vi "IO配置检测.vi"(7 "错误输入（无错误）":errorcluster, 8 "配置检索操作":T11, 9 "点动轴选择":T10=enum."出料轴", 10 "输出控制":T6, 11 "输入读取":T1) -> (0 "输出配置提取集合":T12, 1 "输入配置提取集合":T12, 3 "轴名称数组":string[](array[string]), 5 "error out":errorcluster)   [LabVIEW 2017]
panel:
  in  "选项卡控件":enum32{"选项卡 1", "选项卡 2", "选项卡 3"}(tab)
  out "轴信息检索list":string[](array[string])
  out "Input检索list":string[](array[string])
  out "Output检索list":string[](array[string])
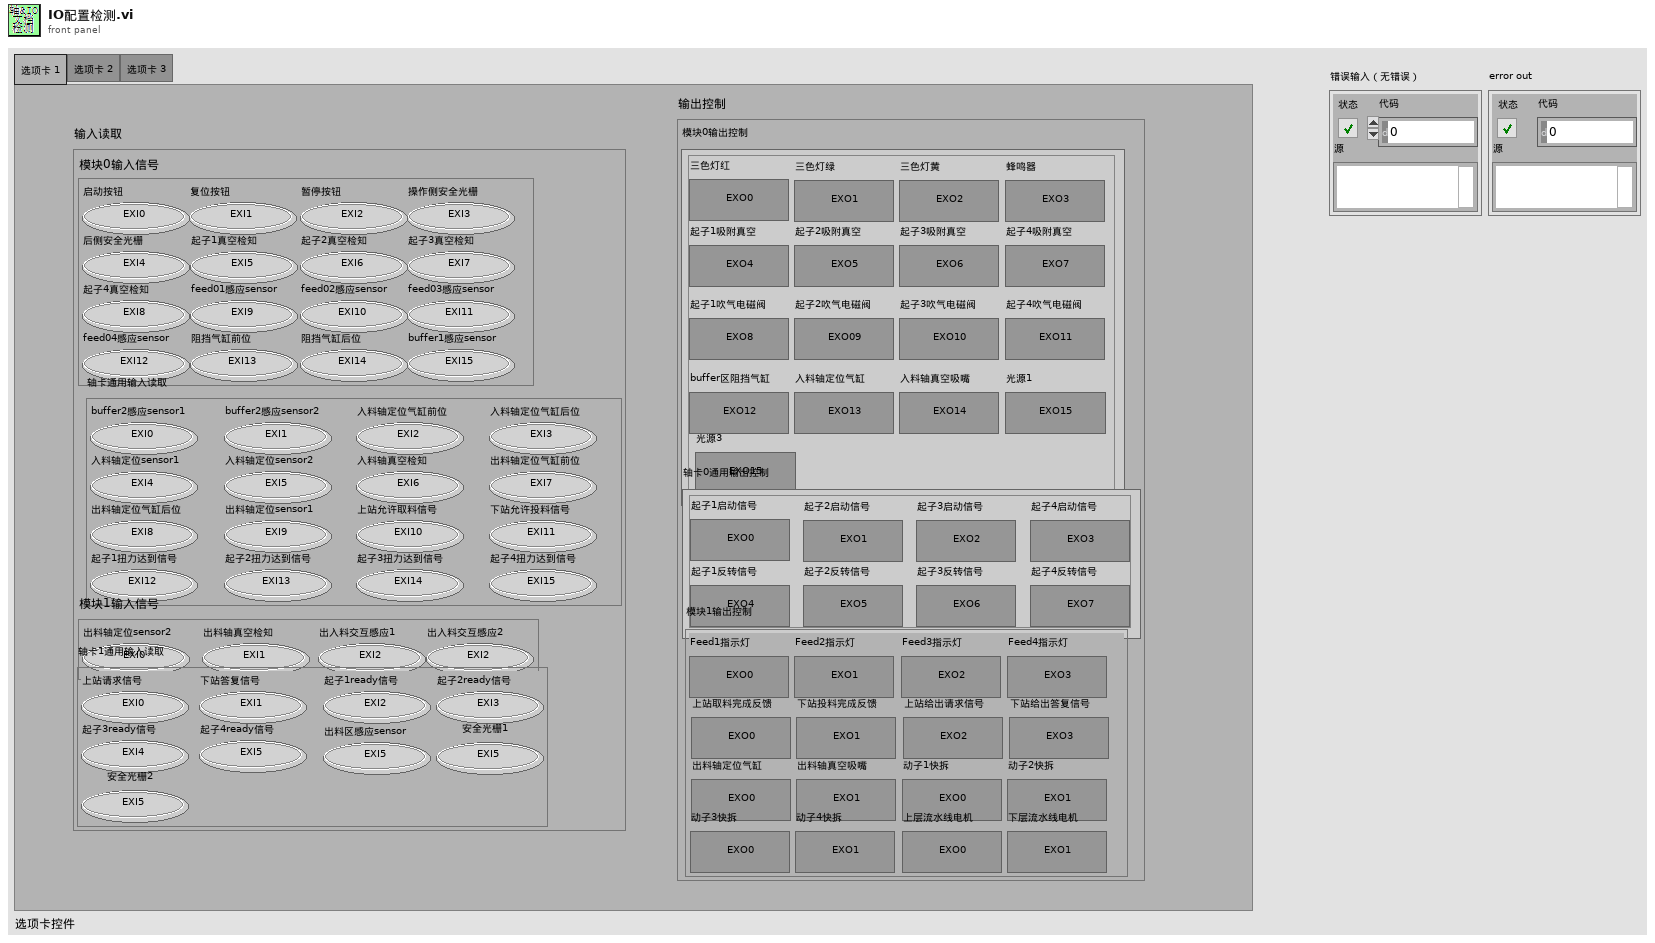
[diagram p1: front panel]
types:
  T1 = typedef "输入读取.ctl" = cluster{"模块0输入信号":T2, "轴卡通用输入读取":T3, "模块1输入信号":T4, "轴卡1通用输入读取":T5}
  T2 = typedef "模块0输入读取.ctl" = cluster{"启动按钮":bool, "复位按钮":bool, "暂停按钮":bool, "操作侧安全光栅":bool, "后侧安全光栅":bool, "起子1真空检知":bool, "起子2真空检知":bool, "起子3真空检知":bool, "起子4真空检知":bool, "feed01感应sensor":bool, "feed02感应sensor":bool, "feed03感应sensor":bool, "feed04感应sensor":bool, "阻挡气缸前位":bool, "阻挡气缸后位":bool, "buffer1感应sensor":bool}
  T3 = typedef "轴卡0通用输入读取.ctl" = cluster{"buffer2感应sensor1":bool, "buffer2感应sensor2":bool, "入料轴定位气缸前位":bool, "入料轴定位气缸后位":bool, "入料轴定位sensor1":bool, "入料轴定位sensor2":bool, "入料轴真空检知":bool, "出料轴定位气缸前位":bool, "出料轴定位气缸后位":bool, "出料轴定位sensor1":bool, "上站允许取料信号":bool, "下站允许投料信号":bool, "起子1扭力达到信号":bool, "起子2扭力达到信号":bool, "起子3扭力达到信号":bool, "起子4扭力达到信号":bool}
  T4 = typedef "模块1输入读取.ctl" = cluster{"出料轴定位sensor2":bool, "出料轴真空检知":bool, "出入料交互感应1":bool, "出入料交互感应2":bool}
  T5 = typedef "轴卡1通用输入读取.ctl" = cluster{"上站请求信号":bool, "下站答复信号":bool, "起子1ready信号":bool, "起子2ready信号":bool, "起子3ready信号":bool, "起子4ready信号":bool, "出料区感应sensor":bool, "安全光栅1":bool, "安全光栅2":bool}
  T6 = typedef "输出控制.ctl" = cluster{"模块0输出控制":T7, "轴卡0通用输出控制":T8, "模块1输出控制":T9}
  T7 = typedef "模块0输出控制.ctl" = cluster{"三色灯红":bool, "三色灯绿":bool, "三色灯黄":bool, "蜂鸣器":bool, "起子1吸附真空":bool, "起子2吸附真空":bool, "起子3吸附真空":bool, "起子4吸附真空":bool, "起子1吹气电磁阀":bool, "起子2吹气电磁阀":bool, "起子3吹气电磁阀":bool, "起子4吹气电磁阀":bool, "buffer区阻挡气缸":bool, "入料轴定位气缸":bool, "入料轴真空吸嘴":bool, "光源1":bool, "光源3":bool}
  T8 = typedef "轴卡0通用输出控制.ctl" = cluster{"起子1启动信号":bool, "起子2启动信号":bool, "起子3启动信号":bool, "起子4启动信号":bool, "起子1反转信号":bool, "起子2反转信号":bool, "起子3反转信号":bool, "起子4反转信号":bool}
  T9 = typedef "模块1输出控制.ctl" = cluster{"Feed1指示灯":bool, "Feed2指示灯":bool, "Feed3指示灯":bool, "Feed4指示灯":bool, "上站取料完成反馈":bool, "下站投料完成反馈":bool, "上站给出请求信号":bool, "下站给出答复信号":bool, "出料轴定位气缸":bool, "出料轴真空吸嘴":bool, "动子1快拆":bool, "动子2快拆":bool, "动子3快拆":bool, "动子4快拆":bool, "上层流水线电机":bool, "下层流水线电机":bool}
  T10 = typedef "轴命名.ctl" = enum16{"入料轴", "出料轴", "动子1轴", "动子2轴", "动子3轴", "动子4轴", "Z轴1号", "Z轴2号", "Z轴3号", "Z轴4号", "driver01", "driver02", "driver03", "driver04"}
  T11 = typedef "配置检索操作.ctl" = enum16{"配置检索", "名称提取", "寄存器提取"}
  T12 = typedef "输入&输出配置提取集合.ctl" = cluster{"IO配置名称":string[], "IO配置点位地址":string[], "IO配置名称索引":i32[], "取反信息":i32[], "簇属性集合":string[]}
  T13 = typedef "文档集合.ctl" = cluster{"固定点位信息":string[][], "轴配置信息":string[][], "动子1&2锁附扭力及检测信息":string[][], "动子3&4锁附扭力及检测信息":string[][], "动子1&2锁附图面坐标信息":string[][], "动子3&4锁附图面坐标信息":string[][], "动子1&2基准拍照参数":string[][], "动子3&4基准拍照参数":string[][], "出入料轴位置信息":string[][], "IO配置信息-Input":string[][], "IO配置信息-Output":string[][]}
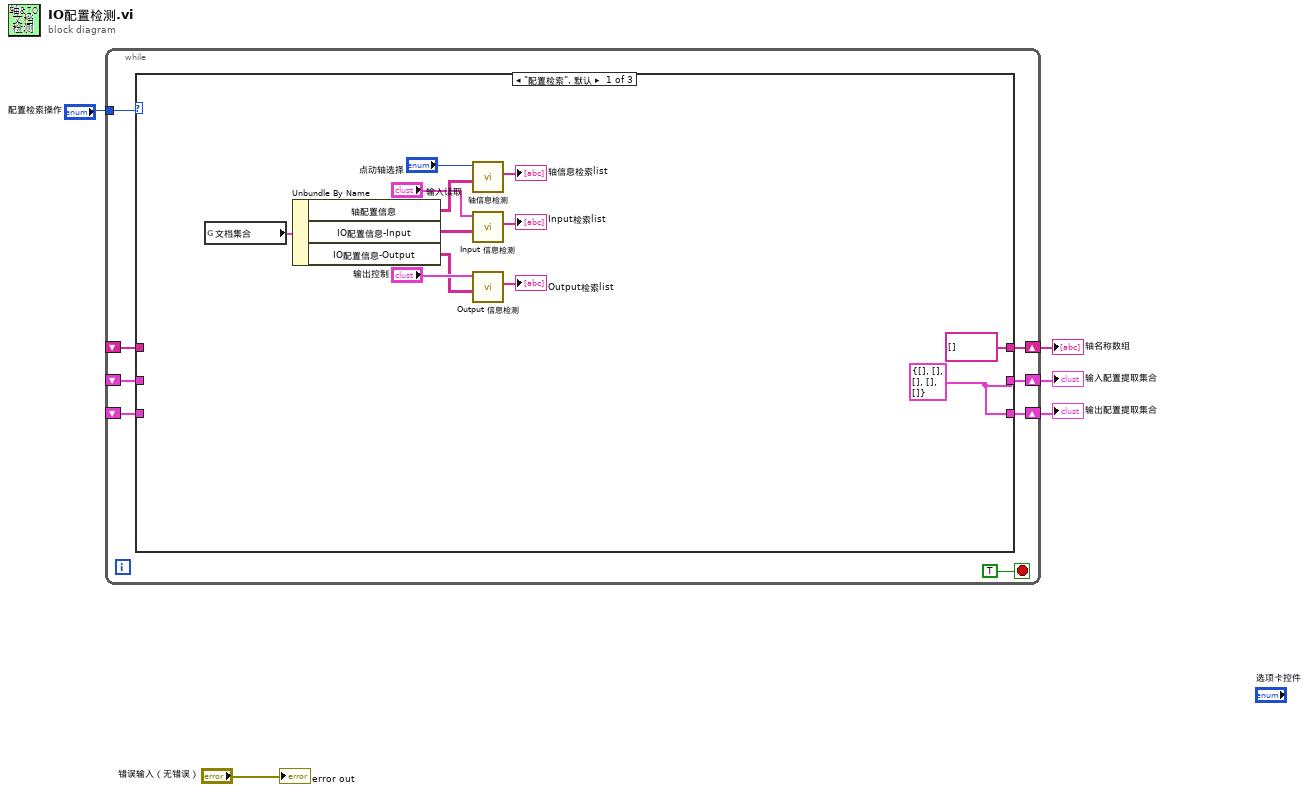
[diagram p0: block diagram]
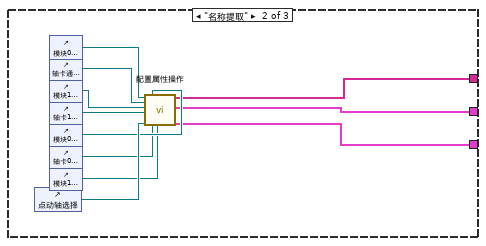
[diagram p2: hidden frame]
diagram:
  n1 = while {
    tunnel: "配置检索操作" -> [w12]
    shift-right: [w11] -> w3
    shift-left: _ -> [w8]
    shift-right: [w10] -> w2
    shift-left: _ -> [w7]
    shift-right: [w9] -> w1
    shift-left: _ -> [w6]
    stop <- TRUE stop-if-true
    n2 = case shown="\"配置检索\", 默认" w12 {
      tunnel: [string[] [] ("轴名称数组") w28 w39] -> w11
      tunnel: [w14 w27 w38] -> w10
      tunnel: [w14 w26 w37] -> w9
      tunnel: w8 -> [_ _ w39]
      tunnel: w7 -> [_ _ w38]
      tunnel: w6 -> [_ _ w37]
      frame "配置检索", Default {
        w14 = T12 {"IO配置名称"=[], "IO配置点位地址"=[], "IO配置名称索引"=[], "取反信息"=[], "簇属性集合"=[]} ("输入配置提取集合")
        n3 = global read "参数全局.vi" "文档集合"() -> (w16:T13)
        n4 = Unbundle By Name(w16) -> ("轴配置信息"=w24:string[][], "IO配置信息-Input"=w23:string[][], "IO配置信息-Output"=w20:string[][])
        n5 = call "轴信息检测.vi"("轴配置信息"=w24, "点动轴选择"="点动轴选择") -> ("轴信息ERROR"=→"轴信息检索list":string[])  [unwired: 9 in]
        n6 = call "Input 信息检测.vi"("Input 配置信息"=w23, "输入读取"="输入读取") -> ("Input  ERROR"=→"Input检索list":string[])  [unwired: 9 in]
        n7 = call "Output 信息检测.vi"("Output配置信息"=w20, "输出控制"="输出控制") -> ("Output Error"=→"Output检索list":string[])  [unwired: 9 in]
      }
      frame "名称提取" {
        n8 = control-ref of="点动轴选择"() -> (w32:refnum<vi>)
        n9 = control-ref of="模块0输入信号"() -> (w36:refnum<vi>)
        n10 = control-ref of="轴卡通用输入读取"() -> (w35:refnum<vi>)
        n11 = control-ref of="模块1输入信号"() -> (w34:refnum<vi>)
        n12 = control-ref of="轴卡1通用输入读取"() -> (w33:refnum<vi>)
        n13 = control-ref of="模块0输出控制"() -> (w31:refnum<vi>)
        n14 = control-ref of="轴卡0通用输出控制"() -> (w30:refnum<vi>)
        n15 = control-ref of="模块1输出控制"() -> (w29:refnum<vi>)
        n16 = call "配置属性操作.vi"("模块0输入信号"=w36, "轴卡通用输入读取"=w35, "模块1输入信号"=w34, "轴卡1通用输入读取"=w33, "轴选择"=w32, "模块0输出控制"=w31, "轴卡0通用输出控制"=w30, "模块1输出控制"=w29) -> ("轴名称数组"=w28:string[], "输入配置提取集合"=w27:T12, "输出配置提取集合"=w26:T12)  [unwired: 9 in]
      }
      frame "寄存器提取" {
      }
    }
  }
  "轴名称数组" <- w3
  "输入配置提取集合" <- w2
  "输出配置提取集合" <- w1
  "error out" <- "错误输入（无错误）"
